vi "Set IO Out State.vi"(8 "error in (no error)":errorcluster, 10 "state":u8, 11 "channel":u8) -> (0 "error out":errorcluster)   [LabVIEW 2021, in "vmmso.lvlib"]
doc: "DLL_API void WINAPI SetIOOutState(unsigned char channel, unsigned char state);"
uses:
  vmmso.lvlib
  vmmso.dll
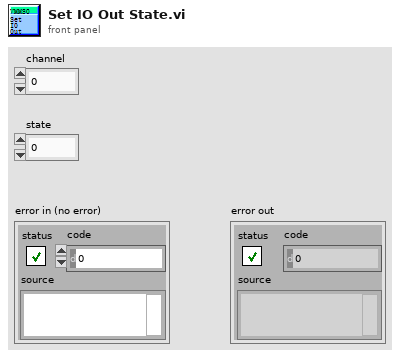
[diagram p1: front panel]
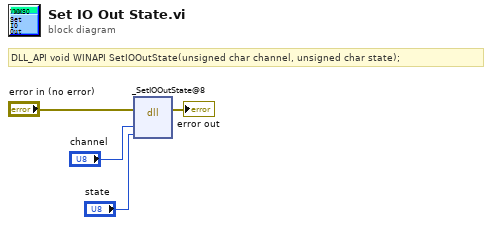
[diagram p0: block diagram]
diagram:
  # "DLL_API void WINAPI SetIOOutState(unsigned char channel, unsigned char state);"
  n1 = dll-call lib="O:/MSO/library/demo-Labview/vmmso/vmmso.*" fn="_SetIOOutState@8"(error in="error in (no error)", "channel"="channel", "state"="state") -> (error out=→"error out":errorcluster)  [unwired: 5 in, 1 out]
